vi "Initialize.vi"(8 "error in (no error)":errorcluster, 10 "Variant":variant, 11 "Thorlabs_PM100D in":refnum<class "Thorlabs_PM100D.lvclass">) -> (0 "error out":errorcluster, 3 "Thorlabs_PM100D out":refnum<class "Thorlabs_PM100D.lvclass">)   [LabVIEW 2020, in "Thorlabs_PM100D.lvclass"]
uses:
  <instrlib>/Classes/Powermeter/Thorlabs_PM100D/Thorlabs_PM100D.lvclass
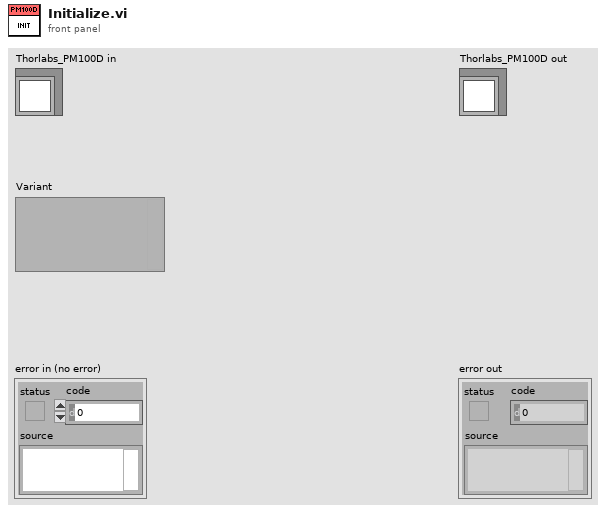
[diagram p1: front panel]
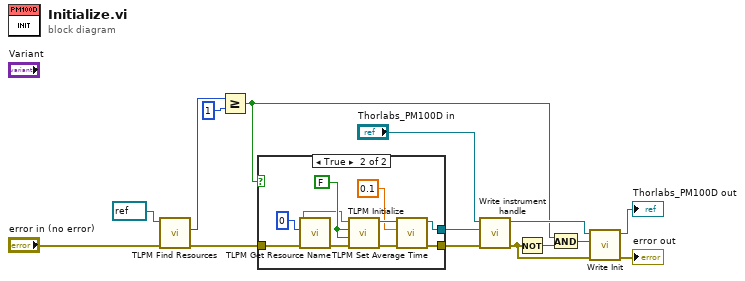
[diagram p0: block diagram]
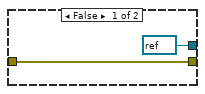
[diagram p2: hidden frame]
diagram:
  n1 = call <instrlib>:"TLPM Find Resources.vi"("error in (no error)"="error in (no error)", "instrument handle"=refnum<visa-resource-name> refnum) -> ("error out"=w12:errorcluster, "Resource Count"=w14:u32)  [unwired: 7 in, 1 out]
  n2 = Greater Or Equal?(x=w14, y=u32 1) -> (x >= y?=w6:bool)
  n3 = case shown="True" w6 {
    tunnel: w12 -> [w17 w23]
    tunnel: [w17 w20] -> w5
    tunnel: [refnum<visa-resource-name> refnum ("instrument handle out") w19] -> w10
    frame False {
    }
    frame True {
      w25 = FALSE ("ID Query (Do Query)")
      n4 = call <instrlib>:"TLPM Get Resource Name.vi"("error in (no error)"=w23, "Index (0)"=u32 0 ("Device Index")) -> ("error out"=w27:errorcluster, "Resource Name"=w24:string)  [unwired: 7 in, 1 out]
      n5 = call <instrlib>:"TLPM Initialize.vi"("error in (no error)"=w27, "Reset Device (Reset Device)"=w25, "ID Query (Do Query)"=w25, "resource name"=w24) -> ("error out"=w22:errorcluster, "instrument handle out"=w21:refnum<visa-resource-name>)  [unwired: 6 in]
      n6 = call <instrlib>:"TLPM Set Average Time.vi"("error in (no error)"=w22, "Average Time (0.0)"=0.1, "instrument handle"=w21) -> ("error out"=w20:errorcluster, "instrument handle out"=w19:refnum<visa-resource-name>)  [unwired: 7 in]
    }
  }
  n7 = call-dynamic "Write instrument handle.vi"("error in (no error)"=w5, "instrument handle"=w10, "Thorlabs_PM100D in"="Thorlabs_PM100D in") -> ("error out"=w3:errorcluster, "Thorlabs_PM100D out"=w8:refnum<class "Thorlabs_PM100D.lvclass">)  [unwired: 7 in]
  n8 = Not(x=w3) -> (.not. x?=w2:bool)
  n9 = And(x=w6, y=w2) -> (x .and. y?=w4:bool)
  n10 = call-dynamic "Write Init.vi"("error in (no error)"=w3, "Init"=w4, "Thorlabs_PM100D in"=w8) -> ("error out"=→"error out":errorcluster, "Thorlabs_PM100D out"=→"Thorlabs_PM100D out":refnum<class "Thorlabs_PM100D.lvclass">)  [unwired: 7 in]
